vi "Instrument Download Waveform.vi"(0 "RFSG handle":refnum<k15>, 5 "Waveform In":T1={"Waveform Name"="Wfm", "Waveform"={"x0"=0.0, "dx"=0.0, "y"=[]}, "Signal Bandwidth (Hz)"=0.0, "PAPR (dB)"=0.0, "Burst Length (s)"=0.0, "Sample Rate"=0.0, "Burst Start Locations"=[], "Burst Stop Locations"=[], "Idle Duration Present?"=FALSE} {"Sample Rate" format="%#_6p"; "Burst Length (s)" format="%#_6p"; "PAPR (dB)" format="%.2f"; "Signal Bandwidth (Hz)" format="%.2f"; "Waveform"."y" format="%.2f"; "Waveform"."dx" format="%^.2e"; "Waveform"."x0" format="%^.2e"}, 11 "error in (no error)":errorcluster) -> (4 "RFSG handle out":refnum<k15>, 15 "error out":errorcluster)   [LabVIEW 2018, in "SG.lvlib"]
uses:
  SG.lvlib
  Typedefs/Waveform.ctl
  <instrlib>/niRFSG/niRFSG.llb/niRFSG Write Arb Waveform (Complex Input SGL).vi
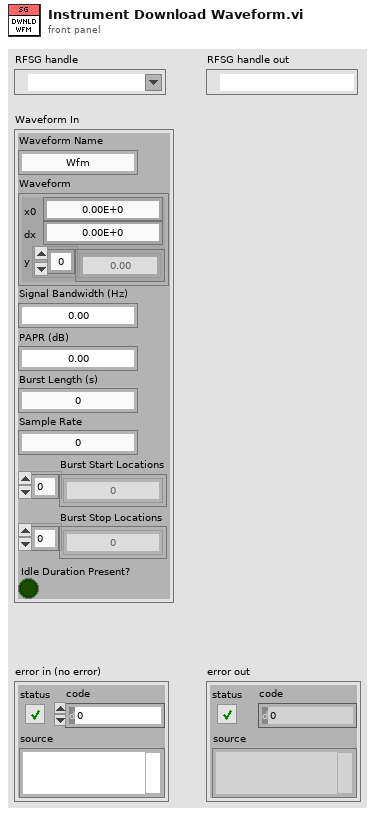
[diagram p1: front panel]
types:
  T1 = typedef "SG.lvlib/Waveform.ctl" = cluster{"Waveform Name":string, "Waveform":cluster{"x0":dbl, "dx":dbl, "y":csg[]}, "Signal Bandwidth (Hz)":dbl, "PAPR (dB)":dbl, "Burst Length (s)":dbl, "Sample Rate":dbl, "Burst Start Locations":i32[], "Burst Stop Locations":i32[], "Idle Duration Present?":bool}
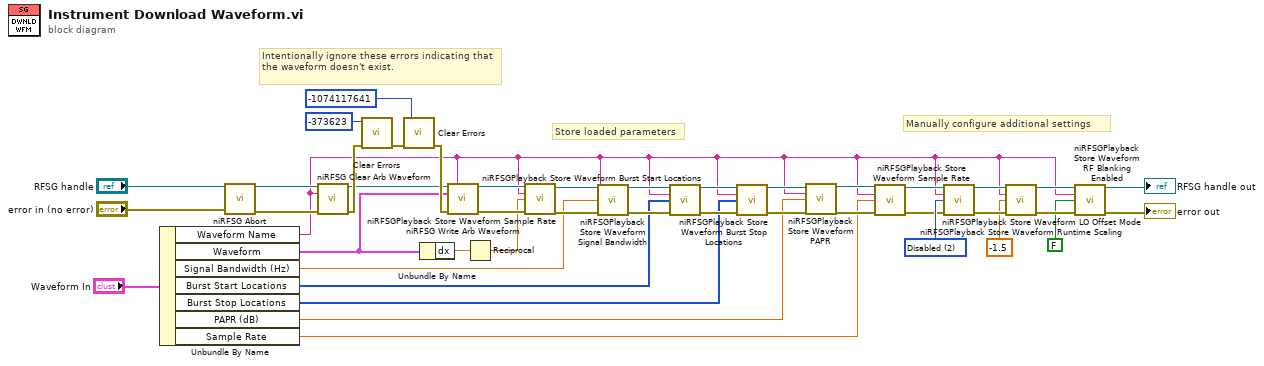
[diagram p0: block diagram]
diagram:
  w25 = 2 items=["Auto", "No Offset", "Disabled"] ("LO offset mode")
  # "Manually configure additional settings"
  # "Store loaded parameters"
  # "Intentionally ignore these errors indicating that the waveform doesn't exist."
  n1 = Unbundle By Name("Waveform In") -> ("Waveform Name"=w2:string, "Waveform"=w23:cluster{"x0":dbl, "dx":dbl, "y":csg[]}, "Signal Bandwidth (Hz)"=w20:dbl, "Burst Start Locations"=w16:i32[], "Burst Stop Locations"=w12:i32[], "PAPR (dB)"=w11:dbl, "Sample Rate"=w1:dbl)
  n2 = call <instrlib>:"niRFSG Abort.vi"("instrument handle"="RFSG handle", "error in"="error in (no error)") -> ("instrument handle out"=w22:refnum<k15>, "error out"=w35:errorcluster)  [unwired: 12 in]
  n3 = call <instrlib>:"niRFSG Clear Arb Waveform.vi"("instrument handle"=w22, "name"=w2, "error in"=w35) -> ("instrument handle out"=w21:refnum<k15>, "error out"=w34:errorcluster)  [unwired: 11 in]
  n4 = call <vilib>:"Clear Errors.vi"("error in (no error)"=w34, "specific error code to clear (0: all)"=-373623) -> ("error out"=w38:errorcluster)  [unwired: 4 in, 1 out]
  n5 = call <vilib>:"Clear Errors.vi"("error in (no error)"=w38, "specific error code to clear (0: all)"=-1074117641) -> ("error out"=w37:errorcluster)  [unwired: 4 in, 1 out]
  n6 = Unbundle By Name(w23) -> ("dx"=w24:dbl)
  n7 = call-poly <instrlib>:"niRFSG Write Arb Waveform.vi"("instrument handle"=w21, "name"=w2, "IQ waveform"=w23, "error in"=w37) -> ("instrument handle out"=w32:refnum<k15>, "error out"=w42:errorcluster)  [unwired: 10 in]
  n8 = Reciprocal(x=w24) -> (1/x=w31:dbl)
  n9 = call <instrlib>:"niRFSGPlayback Store Waveform Sample Rate.vi"("instrument handle in"=w32, "waveform name"=w2, "sample rate"=w31, "error in"=w42) -> ("instrument handle out"=w28:refnum<k15>, "error out"=w40:errorcluster)  [unwired: 10 in]
  n10 = call <instrlib>:"niRFSGPlayback Store Waveform Signal Bandwidth.vi"("instrument handle in"=w28, "waveform name"=w2, "signal bandwidth"=w20, "error in"=w40) -> ("instrument handle out"=w17:refnum<k15>, "error out"=w36:errorcluster)  [unwired: 10 in]
  n11 = call <instrlib>:"niRFSGPlayback Store Waveform Burst Start Locations.vi"("instrument handle in"=w17, "waveform name"=w2, "burst start locations"=w16, "error in"=w36) -> ("instrument handle out"=w14:refnum<k15>, "error out"=w18:errorcluster)  [unwired: 10 in]
  n12 = call <instrlib>:"niRFSGPlayback Store Waveform Burst Stop Locations.vi"("instrument handle in"=w14, "waveform name"=w2, "burst stop locations"=w12, "error in"=w18) -> ("instrument handle out"=w13:refnum<k15>, "error out"=w15:errorcluster)  [unwired: 10 in]
  n13 = call <instrlib>:"niRFSGPlayback Store Waveform PAPR.vi"("instrument handle in"=w13, "waveform name"=w2, "PAPR"=w11, "error in"=w15) -> ("instrument handle out"=w4:refnum<k15>, "error out"=w39:errorcluster)  [unwired: 10 in]
  n14 = call <instrlib>:"niRFSGPlayback Store Waveform Sample Rate.vi"("instrument handle in"=w4, "waveform name"=w2, "sample rate"=w1, "error in"=w39) -> ("instrument handle out"=w3:refnum<k15>, "error out"=w5:errorcluster)  [unwired: 10 in]
  n15 = call <instrlib>:"niRFSGPlayback Store Waveform LO Offset Mode.vi"("instrument handle in"=w3, "waveform name"=w2, "LO offset mode"=w25, "error in"=w5) -> ("instrument handle out"=w29:refnum<k15>, "error out"=w41:errorcluster)  [unwired: 10 in]
  n16 = call <instrlib>:"niRFSGPlayback Store Waveform Runtime Scaling.vi"("instrument handle in"=w29, "waveform name"=w2, "runtime scaling"=-1.5, "error in"=w41) -> ("instrument handle out"=w8:refnum<k15>, "error out"=w10:errorcluster)  [unwired: 10 in]
  n17 = call <instrlib>:"niRFSGPlayback Store Waveform RF Blanking Enabled.vi"("instrument handle in"=w8, "waveform name"=w2, "RF blanking enabled"=FALSE, "error in"=w10) -> ("instrument handle out"=→"RFSG handle out":refnum<k15>, "error out"=→"error out":errorcluster)  [unwired: 10 in]
